vi "Create Resource in Controls and Wire Unbundler - Multiple Converter.vi"(0 "node in":refnum<vi>, 5 "unbundle output term":refnum<vi>[](array[refnum]), 11 "error in":errorcluster) -> (15 "error out":errorcluster)   [LabVIEW 2021, in "Converter.lvlib"]
uses:
  Converter.lvlib
  Converter Reusables/Converter Reusables.lvlib
  Path Functions/Path Functions.lvlib
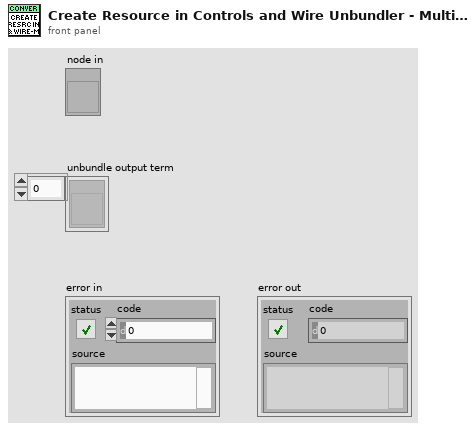
[diagram p1: front panel]
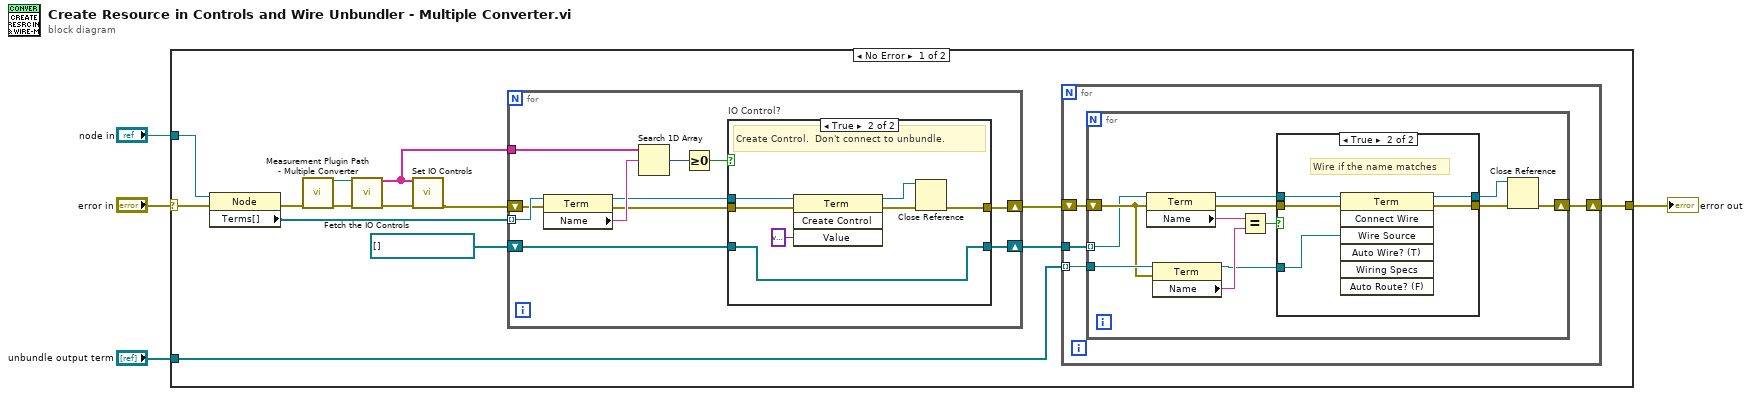
[diagram p0: block diagram]
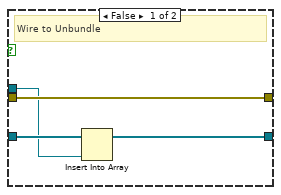
[diagram p3: hidden frame]
diagram:
  n1 = case shown="No Error" "error in" {
    selector: "error in" -> [w16 w64]
    tunnel: [w9 w64] -> w3
    tunnel: "unbundle output term" -> [w18 _]
    tunnel: "node in" -> [w17 _]
    frame No Error {
      n2 = property class="Node"(reference=w17, error in=w16) -> (error out=w6:errorcluster, "Terms[]"=w11:refnum<vi>[])  [unwired: 1 out]
      n3 = call "Measurement Plugin Path - Multiple Converter.vi"("error in"=w6) -> ("new code module"=w7:path, "error out"=w5:errorcluster)  [unwired: 2 in, 11 out]
      n4 = call "Fetch the IO Controls.vi"("vi path"=w7, "error in"=w5) -> ("io controls[]"=w14:string[], "error out"=w15:errorcluster)  [unwired: 12 in]
      n5 = call "Set IO Controls.vi"("io controls[]"=w14, "error in"=w15) -> ("error out"=w12:errorcluster)  [unwired: 13 in]
      n6 = for {
        tunnel: w11 -> [w52] mode=indexing
        tunnel: w14 -> [w49]
        shift-right: [w44] -> w10
        shift-left: refnum<vi>[] [] -> [w43]
        shift-right: [w42] -> w13
        shift-left: w12 -> [w51]
        n7 = property class="Term"(reference=w52, error in=w51) -> (reference out=w46:refnum<vi>, error out=w45:errorcluster, "Name"=w48:string)
        n8 = Search 1D Array(1D array=w49, element=w48) -> (index of element=w50:i32)  [unwired: 1 in]
        n9 = Greater Or Equal To 0?(x=w50) -> (x >= 0?=w47:bool)
        n10 = case "IO Control?" shown="True" w47 {
          tunnel: w45 -> [w56 w63]
          tunnel: [w56 w59] -> w42
          tunnel: w46 -> [w53 w60]
          tunnel: [w54 w57] -> w44
          tunnel: w43 -> [w55 w57]
          frame False {
            # "Wire to Unbundle"
            n11 = Insert Into Array(array=w55, new element=w53) -> (w54:refnum<vi>[])  [unwired: 1 in]
          }
          frame True {
            # "Create Control.  Don't connect to unbundle."
            n12 = invoke class="Term" method="Create Control"(reference=w60, error in=w63, "Value"=variant) -> (reference out=w58:refnum<vi>, error out=w62:errorcluster)  [unwired: 1 in, 2 out]
            n13 = Close Reference(reference=w58, error in (no error)=w62) -> (error out=w59:errorcluster)
          }
        }
      }
      n14 = for {
        tunnel: w10 -> [w20]
        tunnel: w18 -> [w19] mode=indexing
        shift-right: [w21] -> w9
        shift-left: w13 -> [w22]
        n15 = for {
          tunnel: w20 -> [w31] mode=indexing
          tunnel: w19 -> [w33]
          shift-right: [w34] -> w21
          shift-left: w22 -> [w32]
          n16 = property class="Term"(reference=w31, error in=w32) -> (reference out=w29:refnum<vi>, error out=w28:errorcluster, "Name"=w24:string)
          n17 = property class="Term"(reference=w33, error in=w32) -> (reference out=w27:refnum<vi>, "Name"=w30:string)  [unwired: 1 out]
          n18 = Equal?(x=w24, y=w30) -> (x = y?=w23:bool)
          n19 = case shown="True" w23 {
            tunnel: w29 -> [w36 w41]
            tunnel: w28 -> [w35 w38]
            tunnel: w27 -> [_ w40]
            tunnel: [w35 w39] -> w26
            tunnel: [w36 w37] -> w25
            frame False {
              # "Ignore"
            }
            frame True {
              # "Wire if the name matches"
              n20 = invoke class="Term" method="Connect Wire"(reference=w41, error in=w38, "Wire Source"=w40) -> (reference out=w37:refnum<vi>, error out=w39:errorcluster)  [unwired: 4 in, 5 out]
            }
          }
          n21 = Close Reference(reference=w25, error in (no error)=w26) -> (error out=w34:errorcluster)
        }
      }
    }
    frame Error {
    }
  }
  "error out" <- w3
